vi "IPC-Modbus-Transfer20150813.vi"(0 "connection ID in":refnum<k5>, 2 "CmdQRef":refnum<queue>, 7 "baud rate (9600)":u32=9600 caption="波特率(9600)", 9 "parity (Even)":u16(ring)=2 caption="奇偶（偶）" items=["无", "奇", "偶"], 11 "错误输入（无错误）":errorcluster) -> (4 "connection ID out":refnum<k5>, 15 "错误输出":errorcluster)   [LabVIEW 2014]
uses:
  Configuration-Global.vi
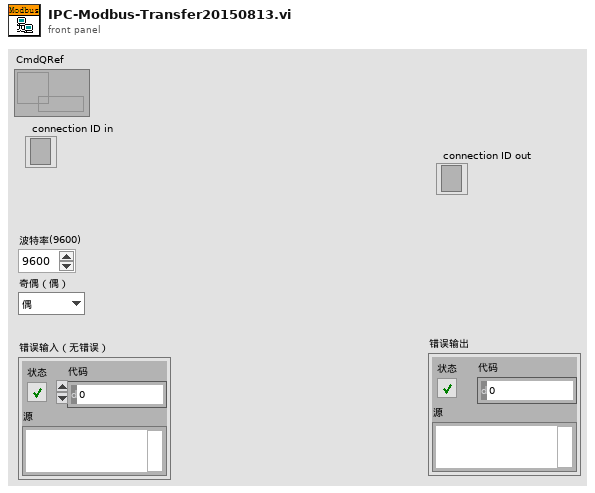
[diagram p1: front panel]
types:
  T1 = cluster{"Transaction ID":u16, "Protocol ID":u16, "Length":u16, " Unit ID":u8}
  T2 = cluster{"Function code":u8, "Starting Address":u16, "Quantity of coils":u16}
  T3 = cluster{"Function code":u8, "Starting Address":u16, "Quantity of inputs":u16}
  T4 = cluster{"Function code":u8, "Starting Address":u16, "Quantity of registers":u16}
  T5 = cluster{"Function code":u8, "Starting Address":u16, "Quantity of input registers":u16}
  T6 = cluster{"Function code":u8, "Output Address":u16, "Output Value":u16}
  T7 = cluster{"Function code":u8, "Register Address":u16, "Register Value":u16}
  T8 = cluster{"Function code":u8, "Starting Address":u16, "Quantity of Outputs":u16, "Byte Count":u8, "Outputs Value":u8[]}
  T9 = cluster{"Function code":u8, "Starting Address":u16, "Quantity of Registers":u16, "Byte Count":u8, "Registers Value":u16[]}
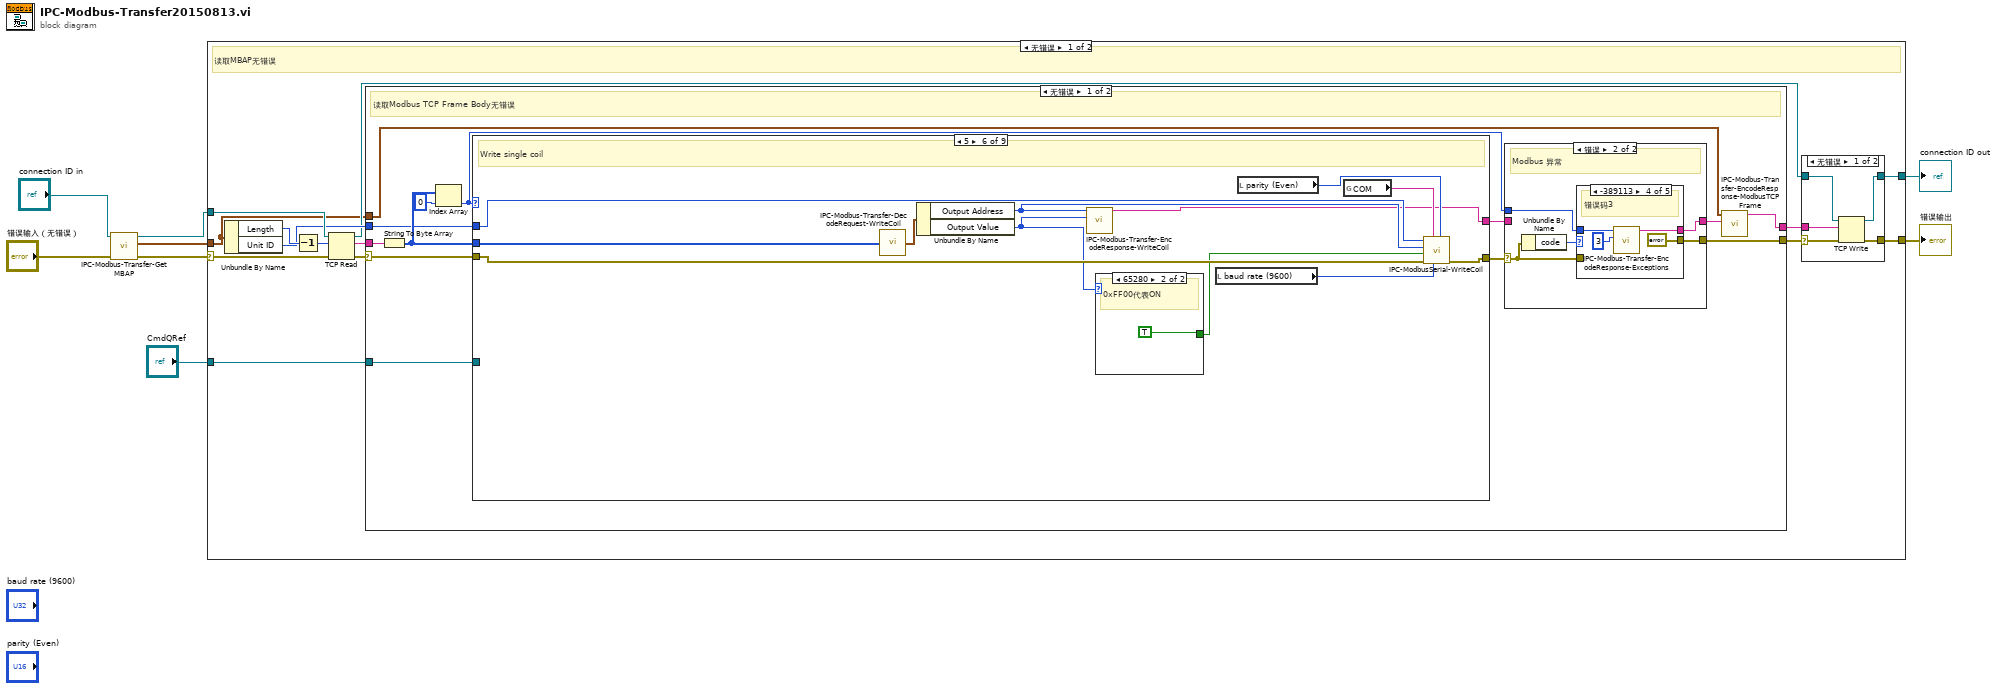
[diagram p0: block diagram]
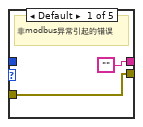
[diagram p3: hidden frame]
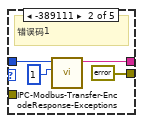
[diagram p4: hidden frame]
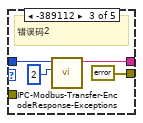
[diagram p5: hidden frame]
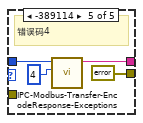
[diagram p6: hidden frame]
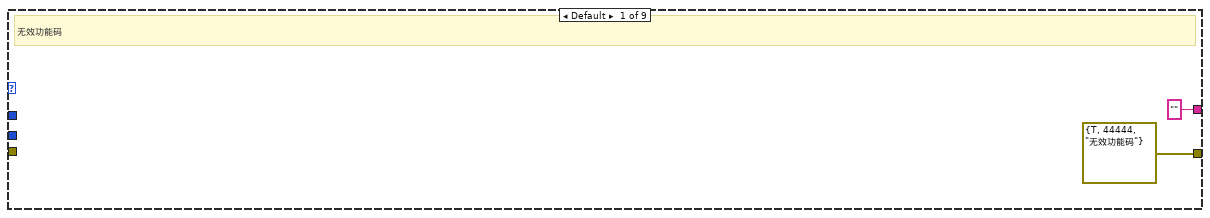
[diagram p7: hidden frame]
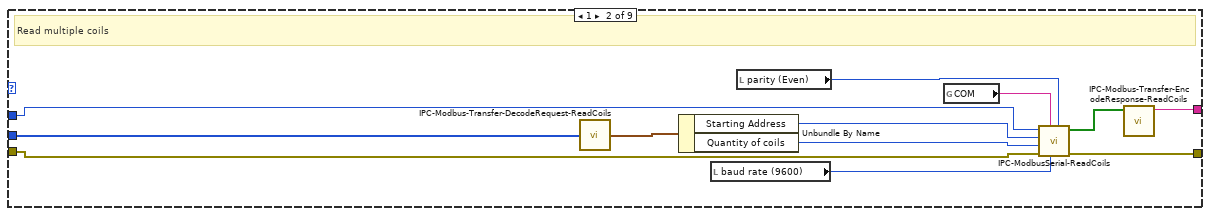
[diagram p8: hidden frame]
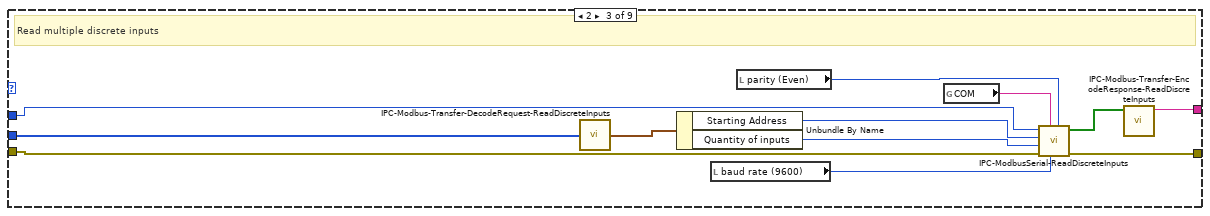
[diagram p9: hidden frame]
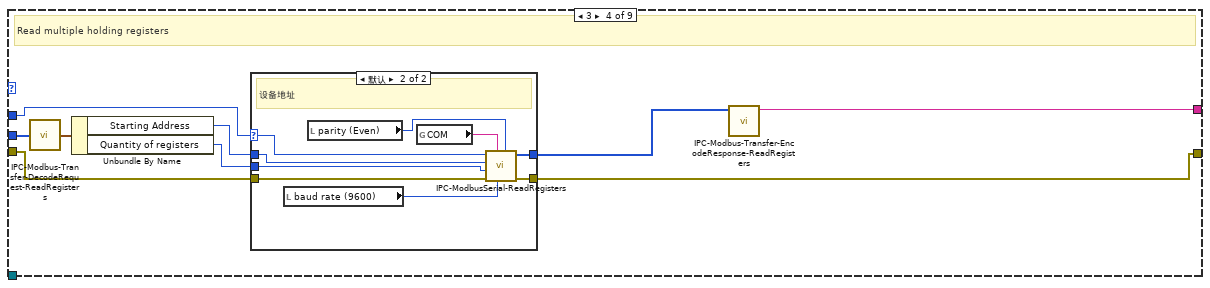
[diagram p10: hidden frame]
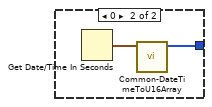
[diagram p12: hidden frame]
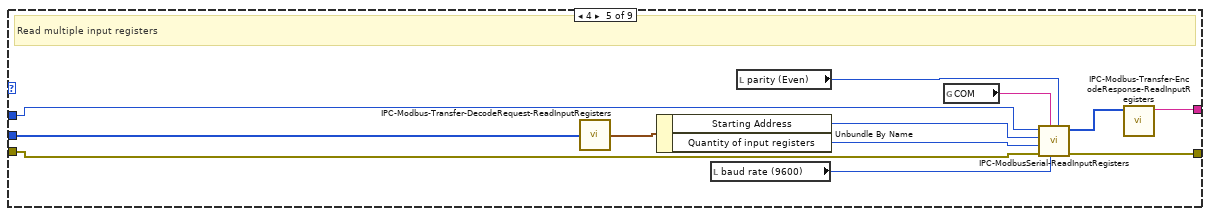
[diagram p13: hidden frame]
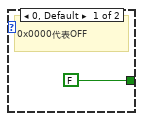
[diagram p14: hidden frame]
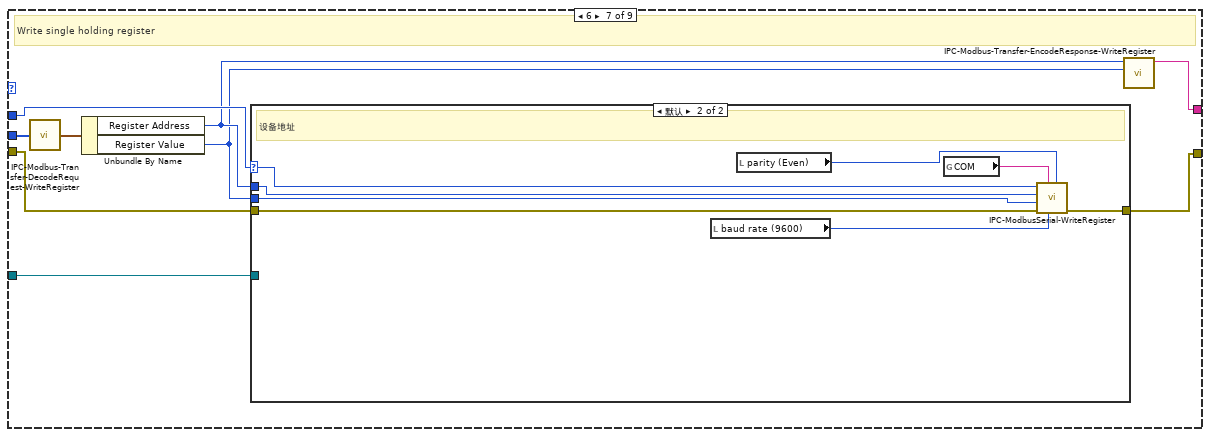
[diagram p15: hidden frame]
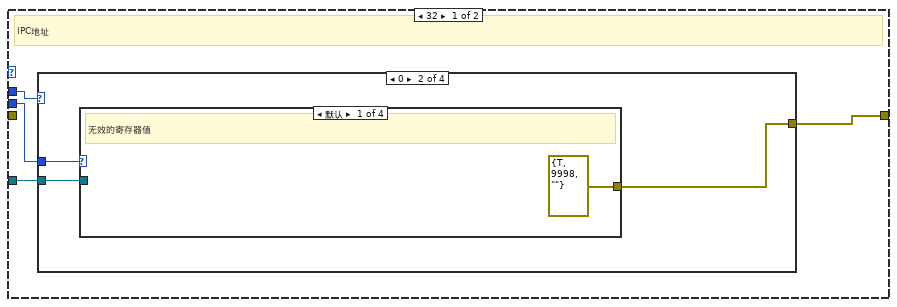
[diagram p16: hidden frame]
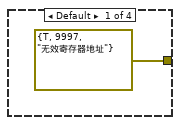
[diagram p17: hidden frame]
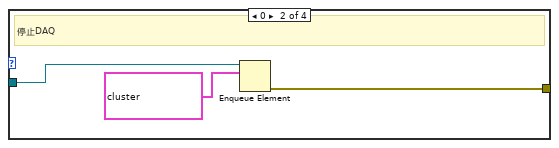
[diagram p18: hidden frame]
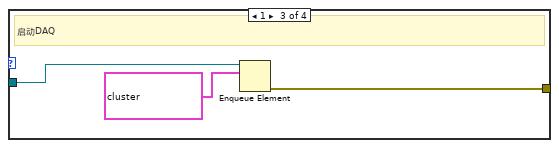
[diagram p19: hidden frame]
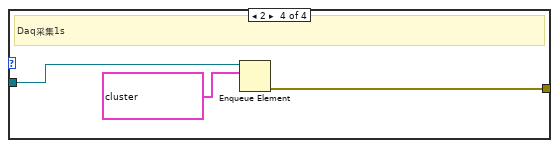
[diagram p20: hidden frame]
diagram:
  n1 = call "IPC-Modbus-Transfer-GetMBAP.vi"("错误输入（无错误）"="错误输入（无错误）", "connection ID in"="connection ID in") -> ("错误输出"=w3:errorcluster, "MBAP"=w1:T1, "连接ID输出"=w2:refnum<k5>)  [unwired: 7 in]
  n2 = case shown="无错误" w3 {
    selector: w3 -> [w19 w205]
    tunnel: w2 -> [w22 w206]
    tunnel: [w21 w206] -> w7
    tunnel: [w20 w205] -> w8
    tunnel: "CmdQRef" -> [w9 _]
    tunnel: w1 -> [w11 _]
    frame No Error {
      # "读取MBAP无错误"
      n3 = Unbundle By Name(w11) -> ("Length"=w18:u16, "Unit ID"=w14:u8)
      n4 = Decrement(x=w18) -> (x-1=w17:u16)
      n5 = TCP Read(connection ID=w22, bytes to read=w17, error in (no error)=w19) -> (connection ID out=w12:refnum<k5>, data out=w16:string, error out=w15:errorcluster)  [unwired: 2 out]
      n6 = case shown="无错误" w15 {
        selector: w15 -> [w32 w197]
        tunnel: w16 -> [w35 _]
        tunnel: [w26 w197] -> w13
        tunnel: w14 -> [w31 _]
        tunnel: w11 -> [w30 _]
        tunnel: [w29 ""] -> w10
        tunnel: w9 -> [w28 _]
        frame No Error {
          # "读取Modbus TCP Frame Body无错误"
          n7 = String To Byte Array(string=w35) -> (unsigned byte array=w33:u8[])
          n8 = Index Array(array=w33, index=0 ("索引")) -> (element=w23:u8)
          n9 = case shown="5" w23 {
            tunnel: w33 -> [_ w74 w79 w95 w112 w133 w142 w177 w189]
            tunnel: w32 -> [_ w72 w78 w93 w113 w130 w143 w178 w191]
            tunnel: w31 -> [_ w66 w80 w90 w114 w131 w141 w179 w190]
            tunnel: [errorcluster {"status"=TRUE, "code"=44444, "source"="无效功能码"} ("错误常量") w64 w75 w89 w110 w124 w139 w174 w187] -> w27
            tunnel: ["" w63 w76 w88 w111 w125 w138 w173 w186] -> w25
            tunnel: w28 -> [_ _ _ _ _ _ w140 _ _]
            frame Default {
              # "无效功能码"
            }
            frame 1 {
              # "Read multiple coils"
              n10 = call "IPC-Modbus-Transfer-DecodeRequest-ReadCoils.vi"("无符号字节数组"=w74) -> ("Read coils request"=w73:T2)  [unwired: 4 in]
              n11 = Unbundle By Name(w73) -> ("Starting Address"=w68:u16, "Quantity of coils"=w67:u16)
              n12 = local read "baud rate (9600)"() -> (w69:u32)
              n13 = local read "parity (Even)"() -> (w70:u16)
              n14 = global read "Configuration-Global.vi" "COM"() -> (w71:string)
              n15 = call "IPC-ModbusSerial-ReadCoils.vi"("parity (Even)"=w70, "baud rate (9600)"=w69, "VISA resource name"=w71, "error in (no error)"=w72, "number of coils"=w67, "starting address"=w68, "unit ID"=w66) -> ("error out"=w64:errorcluster, "coil values"=w65:bool[])  [unwired: 2 in]
              n16 = call "IPC-Modbus-Transfer-EncodeResponse-ReadCoils.vi"("Coil Status"=w65) -> ("输出字符串"=w63:string)  [unwired: 10 in]
            }
            frame 2 {
              # "Read multiple discrete inputs"
              n17 = call "IPC-Modbus-Transfer-DecodeRequest-ReadDiscreteInputs.vi"("无符号字节数组"=w79) -> ("Read discrete inputs request"=w86:T3)  [unwired: 4 in]
              n18 = Unbundle By Name(w86) -> ("Starting Address"=w82:u16, "Quantity of inputs"=w81:u16)
              n19 = local read "baud rate (9600)"() -> (w83:u32)
              n20 = local read "parity (Even)"() -> (w84:u16)
              n21 = global read "Configuration-Global.vi" "COM"() -> (w85:string)
              n22 = call "IPC-ModbusSerial-ReadDiscreteInputs.vi"("parity (Even)"=w84, "baud rate (9600)"=w83, "VISA resource name"=w85, "error in (no error)"=w78, "number of discrete inputs"=w81, "starting address"=w82, "unit ID"=w80) -> ("error out"=w75:errorcluster, "discrete input values"=w77:bool[])  [unwired: 2 in]
              n23 = call "IPC-Modbus-Transfer-EncodeResponse-ReadDiscreteInputs.vi"("Input Status"=w77) -> ("输出字符串"=w76:string)  [unwired: 10 in]
            }
            frame 3 {
              # "Read multiple holding registers"
              n24 = call "IPC-Modbus-Transfer-DecodeRequest-ReadRegisters.vi"("无符号字节数组"=w95) -> ("Read registers request"=w94:T4)  [unwired: 4 in]
              n25 = Unbundle By Name(w94) -> ("Starting Address"=w92:u16, "Quantity of registers"=w91:u16)
              n26 = case shown="默认" w90 {
                selector: w90 -> [_ w101]
                tunnel: w93 -> [w96 w106]
                tunnel: w92 -> [w98 w105]
                tunnel: w91 -> [_ w104]
                tunnel: [w96 w103] -> w89
                tunnel: [w97 w102] -> w87
                frame 32 {
                  # "IPC地址"
                  n27 = case shown="默认" w98 {
                    tunnel: [_ w99] -> w97
                    frame Default {
                    }
                    frame 0 {
                      n28 = Get Date/Time In Seconds() -> (seconds since 1Jan1904=w100:timestamp)
                      n29 = call "Common-DateTimeToU16Array.vi"("时间标识"=w100) -> ("U16Array"=w99:u16[])  [unwired: 10 in]
                    }
                  }
                }
                frame Default {
                  # "设备地址"
                  n30 = local read "baud rate (9600)"() -> (w107:u32)
                  n31 = local read "parity (Even)"() -> (w108:u16)
                  n32 = global read "Configuration-Global.vi" "COM"() -> (w109:string)
                  n33 = call "IPC-ModbusSerial-ReadRegisters.vi"("parity (Even)"=w108, "baud rate (9600)"=w107, "VISA resource name"=w109, "error in (no error)"=w106, "number of holding registers"=w104, "starting address"=w105, "unit ID"=w101) -> ("error out"=w103:errorcluster, "register values"=w102:u16[])  [unwired: 2 in]
                }
              }
              n34 = call "IPC-Modbus-Transfer-EncodeResponse-ReadRegisters.vi"("Register value"=w87) -> ("输出字符串"=w88:string)  [unwired: 10 in]
            }
            frame 4 {
              # "Read multiple input registers"
              n35 = call "IPC-Modbus-Transfer-DecodeRequest-ReadInputRegisters.vi"("无符号字节数组"=w112) -> ("Read input registers request"=w121:T5)  [unwired: 4 in]
              n36 = Unbundle By Name(w121) -> ("Starting Address"=w117:u16, "Quantity of input registers"=w116:u16)
              n37 = local read "baud rate (9600)"() -> (w118:u32)
              n38 = local read "parity (Even)"() -> (w119:u16)
              n39 = global read "Configuration-Global.vi" "COM"() -> (w120:string)
              n40 = call "IPC-ModbusSerial-ReadInputRegisters.vi"("parity (Even)"=w119, "baud rate (9600)"=w118, "VISA resource name"=w120, "error in (no error)"=w113, "number of input registers"=w116, "starting address"=w117, "unit ID"=w114) -> ("error out"=w110:errorcluster, "register values"=w115:u16[])  [unwired: 2 in]
              n41 = call "IPC-Modbus-Transfer-EncodeResponse-ReadInputRegisters.vi"("Input Registers"=w115) -> ("输出字符串"=w111:string)  [unwired: 10 in]
            }
            frame 5 {
              # "Write single coil"
              n42 = call "IPC-Modbus-Transfer-DecodeRequest-WriteCoil.vi"("无符号字节数组"=w133) -> ("Write coil request"=w132:T6)  [unwired: 4 in]
              n43 = Unbundle By Name(w132) -> ("Output Address"=w126:u16, "Output Value"=w123:u16)
              n44 = call "IPC-Modbus-Transfer-EncodeResponse-WriteCoil.vi"("Output Value"=w123, "Output Address"=w126) -> ("输出字符串"=w125:string)  [unwired: 9 in]
              n45 = case shown="65280" w123 {
                tunnel: [FALSE TRUE] -> w122
                frame 0, Default {
                  # "0x0000代表OFF"
                }
                frame 65280 {
                  # "0xFF00代表ON"
                }
              }
              n46 = local read "baud rate (9600)"() -> (w129:u32)
              n47 = local read "parity (Even)"() -> (w127:u16)
              n48 = global read "Configuration-Global.vi" "COM"() -> (w128:string)
              n49 = call "IPC-ModbusSerial-WriteCoil.vi"("parity (Even)"=w127, "baud rate (9600)"=w129, "VISA resource name"=w128, "error in (no error)"=w130, "coil value"=w122, "address"=w126, "unit ID"=w131) -> ("error out"=w124:errorcluster)  [unwired: 4 in]
            }
            frame 6 {
              # "Write single holding register"
              n50 = call "IPC-Modbus-Transfer-DecodeRequest-WriteRegister.vi"("无符号字节数组"=w142) -> ("Write register request"=w144:T7)  [unwired: 4 in]
              n51 = Unbundle By Name(w144) -> ("Register Address"=w137:u16, "Register Value"=w136:u16)
              n52 = case shown="默认" w141 {
                selector: w141 -> [_ w163]
                tunnel: w137 -> [w148 w167]
                tunnel: w143 -> [_ w166]
                tunnel: [w145 w165] -> w139
                tunnel: w136 -> [w147 w164]
                tunnel: w140 -> [w146 _]
                frame 32 {
                  # "IPC地址"
                  n53 = case shown="0" w148 {
                    tunnel: w146 -> [_ w152 _ _]
                    tunnel: w147 -> [_ w151 _ _]
                    tunnel: [errorcluster {"status"=TRUE, "code"=9997, "source"="无效寄存器地址"} ("错误常量") w150 _ _] -> w145
                    frame Default {
                    }
                    frame 0 {
                      n54 = case shown="默认" w151 {
                        tunnel: w152 -> [_ w155 w157 w160]
                        tunnel: [errorcluster {"status"=TRUE, "code"=9998, "source"=""} ("错误常量") w154 w158 w161] -> w150
                        frame Default {
                          # "无效的寄存器值"
                        }
                        frame 0 {
                          # "停止DAQ"
                          n55 = Enqueue Element(queue=w155, element=cluster{"Data":variant, "State":string} {"Data"=variant, "State"="Cmd::StopDaq"} ("元素")) -> (error out=w154:errorcluster)  [unwired: 2 in, 2 out]
                        }
                        frame 1 {
                          # "启动DAQ"
                          n56 = Enqueue Element(queue=w157, element=cluster{"Data":variant, "State":string} {"Data"=variant, "State"="Cmd::StartDaq"} ("元素")) -> (error out=w158:errorcluster)  [unwired: 2 in, 2 out]
                        }
                        frame 2 {
                          # "Daq采集1s"
                          n57 = Enqueue Element(queue=w160, element=cluster{"Data":variant, "State":string} {"Data"=variant, "State"="Cmd::DaqOnce"} ("元素")) -> (error out=w161:errorcluster)  [unwired: 2 in, 2 out]
                        }
                      }
                    }
                    frame 1 {
                      # "设置6133频率"
                    }
                    frame 2 {
                      # "设置6220频率"
                    }
                  }
                }
                frame Default {
                  # "设备地址"
                  n58 = local read "baud rate (9600)"() -> (w170:u32)
                  n59 = local read "parity (Even)"() -> (w168:u16)
                  n60 = global read "Configuration-Global.vi" "COM"() -> (w169:string)
                  n61 = call "IPC-ModbusSerial-WriteRegister.vi"("parity (Even)"=w168, "baud rate (9600)"=w170, "VISA resource name"=w169, "error in (no error)"=w166, "holding register value"=w164, "address"=w167, "unit ID"=w163) -> ("error out"=w165:errorcluster)  [unwired: 4 in]
                }
              }
              n62 = call "IPC-Modbus-Transfer-EncodeResponse-WriteRegister.vi"("Register Value"=w136, "Register Address"=w137) -> ("输出字符串"=w138:string)  [unwired: 9 in]
            }
            frame 15 {
              # "Write multiple coils"
              n63 = call "IPC-Modbus-Transfer-DecodeRequest-WriteMulCoils.vi"("无符号字节数组"=w177) -> ("Write Multiple Coils request"=w183:T8)  [unwired: 4 in]
              n64 = Unbundle By Name(w183) -> ("Starting Address"=w172:u16, "Quantity of Outputs"=w171:u16, "Outputs Value"=w176:u8[])
              n65 = local read "baud rate (9600)"() -> (w182:u32)
              n66 = call "IPC-Modbus-U8ArrayToBitArray.vi"("U8 Array"=w176, "Bit Array size"=w171) -> ("Bit Array"=w175:bool[])  [unwired: 7 in]
              n67 = local read "parity (Even)"() -> (w180:u16)
              n68 = call "IPC-Modbus-Transfer-EncodeResponse-WriteMulCoils.vi"("Quantity of outputs"=w171, "Starting Address"=w172) -> ("输出字符串"=w173:string)  [unwired: 9 in]
              n69 = global read "Configuration-Global.vi" "COM"() -> (w181:string)
              n70 = call "IPC-ModbusSerial-WriteMulCoils.vi"("parity (Even)"=w180, "baud rate (9600)"=w182, "VISA resource name"=w181, "error in (no error)"=w178, "coil values"=w175, "starting address"=w172, "unit ID"=w179) -> ("error out"=w174:errorcluster)  [unwired: 4 in]
            }
            frame 16 {
              # "Write multiple holding registers"
              n71 = call "IPC-Modbus-Transfer-DecodeRequest-WriteMulRegisters.vi"("无符号字节数组"=w189) -> ("Write Multiple Registers request"=w195:T9)  [unwired: 4 in]
              n72 = Unbundle By Name(w195) -> ("Starting Address"=w185:u16, "Quantity of Registers"=w184:u16, "Registers Value"=w188:u16[])
              n73 = local read "baud rate (9600)"() -> (w194:u32)
              n74 = local read "parity (Even)"() -> (w192:u16)
              n75 = global read "Configuration-Global.vi" "COM"() -> (w193:string)
              n76 = call "IPC-Modbus-Transfer-EncodeResponse-WriteMulRegisters.vi"("Quantity of registers"=w184, "Starting Address"=w185) -> ("输出字符串"=w186:string)  [unwired: 9 in]
              n77 = call "IPC-ModbusSerial-WriteMulRegisters.vi"("parity (Even)"=w192, "baud rate (9600)"=w194, "VISA resource name"=w193, "error in (no error)"=w191, "holding register values"=w188, "starting address"=w185, "unit ID"=w190) -> ("error out"=w187:errorcluster)  [unwired: 4 in]
            }
          }
          n78 = case shown="错误" w27 {
            selector: w27 -> [w37 w41]
            tunnel: [w36 w39] -> w24
            tunnel: [w37 w40] -> w26
            tunnel: w23 -> [_ w38]
            tunnel: w25 -> [w36 _]
            frame No Error {
              # "无Modbus异常"
            }
            frame Error {
              # "Modbus 异常"
              n79 = Unbundle By Name(w41) -> ("code"=w42:i32)
              n80 = case shown="-389113" w42 {
                tunnel: w41 -> [w44 _ _ _ _]
                tunnel: [w44 errorcluster {"status"=FALSE, "code"=0, "source"=""} ("错误常量") errorcluster {"status"=FALSE, "code"=0, "source"=""} ("错误常量") errorcluster {"status"=FALSE, "code"=0, "source"=""} ("错误常量") errorcluster {"status"=FALSE, "code"=0, "source"=""} ("错误常量")] -> w40
                tunnel: ["" w47 w51 w55 w59] -> w39
                tunnel: w38 -> [_ w45 w49 w53 w57]
                frame Default {
                  # "非modbus异常引起的错误"
                }
                frame -389111 {
                  # "错误码1"
                  n81 = call "IPC-Modbus-Transfer-EncodeResponse-Exceptions.vi"("错误码"=u8 1, "功能码"=w45) -> ("输出字符串"=w47:string)  [unwired: 9 in]
                }
                frame -389112 {
                  # "错误码2"
                  n82 = call "IPC-Modbus-Transfer-EncodeResponse-Exceptions.vi"("错误码"=u8 2, "功能码"=w49) -> ("输出字符串"=w51:string)  [unwired: 9 in]
                }
                frame -389113 {
                  # "错误码3"
                  n83 = call "IPC-Modbus-Transfer-EncodeResponse-Exceptions.vi"("错误码"=u8 3, "功能码"=w53) -> ("输出字符串"=w55:string)  [unwired: 9 in]
                }
                frame -389114 {
                  # "错误码4"
                  n84 = call "IPC-Modbus-Transfer-EncodeResponse-Exceptions.vi"("错误码"=u8 4, "功能码"=w57) -> ("输出字符串"=w59:string)  [unwired: 9 in]
                }
              }
            }
          }
          n85 = call "IPC-Modbus-Transfer-EncodeResponse-ModbusTCPFrame.vi"("Modbus TCP Frame Body"=w24, "MBAP"=w30) -> ("输出字符串"=w29:string)  [unwired: 9 in]
        }
        frame Error {
          # "读取Modbus TCP Frame Body出错"
        }
      }
      n86 = case shown="无错误" w13 {
        selector: w13 -> [w201 w203]
        tunnel: [w200 w203] -> w20
        tunnel: [w198 w204] -> w21
        tunnel: w12 -> [w199 w204]
        tunnel: w10 -> [w202 _]
        frame No Error {
          n87 = TCP Write(connection ID=w199, data in=w202, error in (no error)=w201) -> (connection ID out=w198:refnum<k5>, error out=w200:errorcluster)  [unwired: 1 in, 1 out]
        }
        frame Error {
        }
      }
    }
    frame Error {
      # "读取MBAP出错"
    }
  }
  "错误输出" <- w8
  "connection ID out" <- w7
